vi "Monitor.vi"() -> ()   [LabVIEW 2018]
uses:
  Global Variables.vi
  <vilib>/Utility/file.llb/Read Delimited Spreadsheet (string).vi
  <vilib>/LVH/i3 JSON/i3-json.lvlib
panel:
  out "String":string
  out "Last Event":string="2:29:04 PM"
  out "Sensors Info":T1(array[cluster])
  out "Instruments":T2(array[cluster])=[{"Name"="Chassis_Sensors.vi", "vi reference"=refnum, "Running?"=FALSE}, {"Name"="PIMAX_1.vi", "vi reference"=refnum, "Running?"=FALSE}, {"Name"="PIMAX_2.vi", "vi reference"=refnum, "Running?"=FALSE}, {"Name"="MotorControl.vi", "vi reference"=refnum, "Running?"=FALSE}, {"Name"="Powermeter_library.lvlib:LV Demo Main.vi", "vi reference"=refnum, "Running?"=FALSE}, {"Name"="Multiplexer.vi", "vi reference"=refnum, "Running?"=FALSE}, {"Name"="NIR.vi", "vi reference"=refnum, "Running?"=FALSE}, {"Name"="Vis.vi", "vi reference"=refnum, "Running?"=FALSE}]
  in  "Add Custom Event":bool
  in  "Custom Event Str":string
  in  "Ring":u16(ring) items=["Proj_VaporTubes", "Proj_H2DT", "Proj_H2DT"]
  in  "Global File Information":T3={"Ring"=0, "SubFolder"="Temp Dependence", "Filename (Meas. Description)"="300C", "Measurement index"=5} {"Ring" items=["Proj_VaporTubes", "Proj_H2DT", "Proj_H2DT"]}
  out "File Size (Mb)":dbl[](array[numeric])
  in  "stop":bool
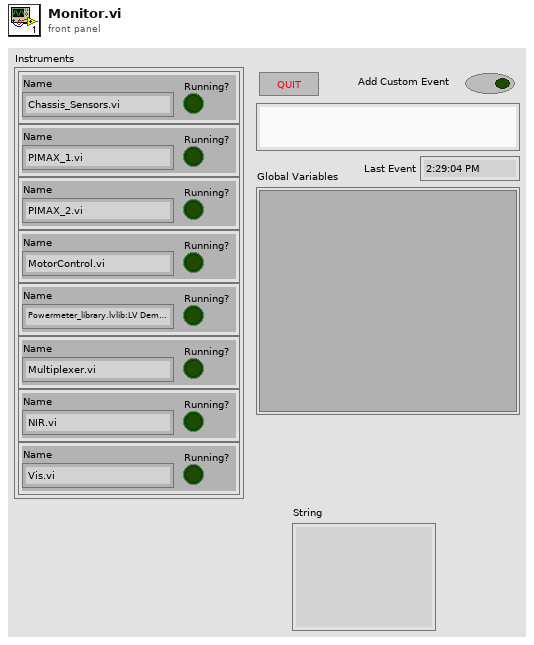
[diagram p1: front panel]
types:
  T1 = cluster{"Label.Text":string, "Panel Ref Out":refnum<vi>, bool}[]
  T2 = cluster{"Name":string, "vi reference":refnum<vi>, "Running?":bool}[]
  T3 = cluster{"Ring":u16, "SubFolder":string, "Filename (Meas. Description)":string, "Measurement index":i32}
  T4 = enum32{"Bad", "Idle", "Run top level", "Running"}
  T5 = cluster{"Name":string, "vi reference":refnum<vi>, bool}
  T6 = cluster{"Name":string, "vi reference":refnum<vi>, bool}[]
  T7 = cluster{"Project":u16, "SubFolder":string, "Filename (Meas. Description)":string, "Measurement index":i32}
  T8 = cluster{"Project 2":u16, "SubFolder 2":string, "Meas. Description 2":string, "Measurement number 2":i32}
  T9 = cluster{"Label.Text":bool, "Panel Ref Out":bool, bool}[]
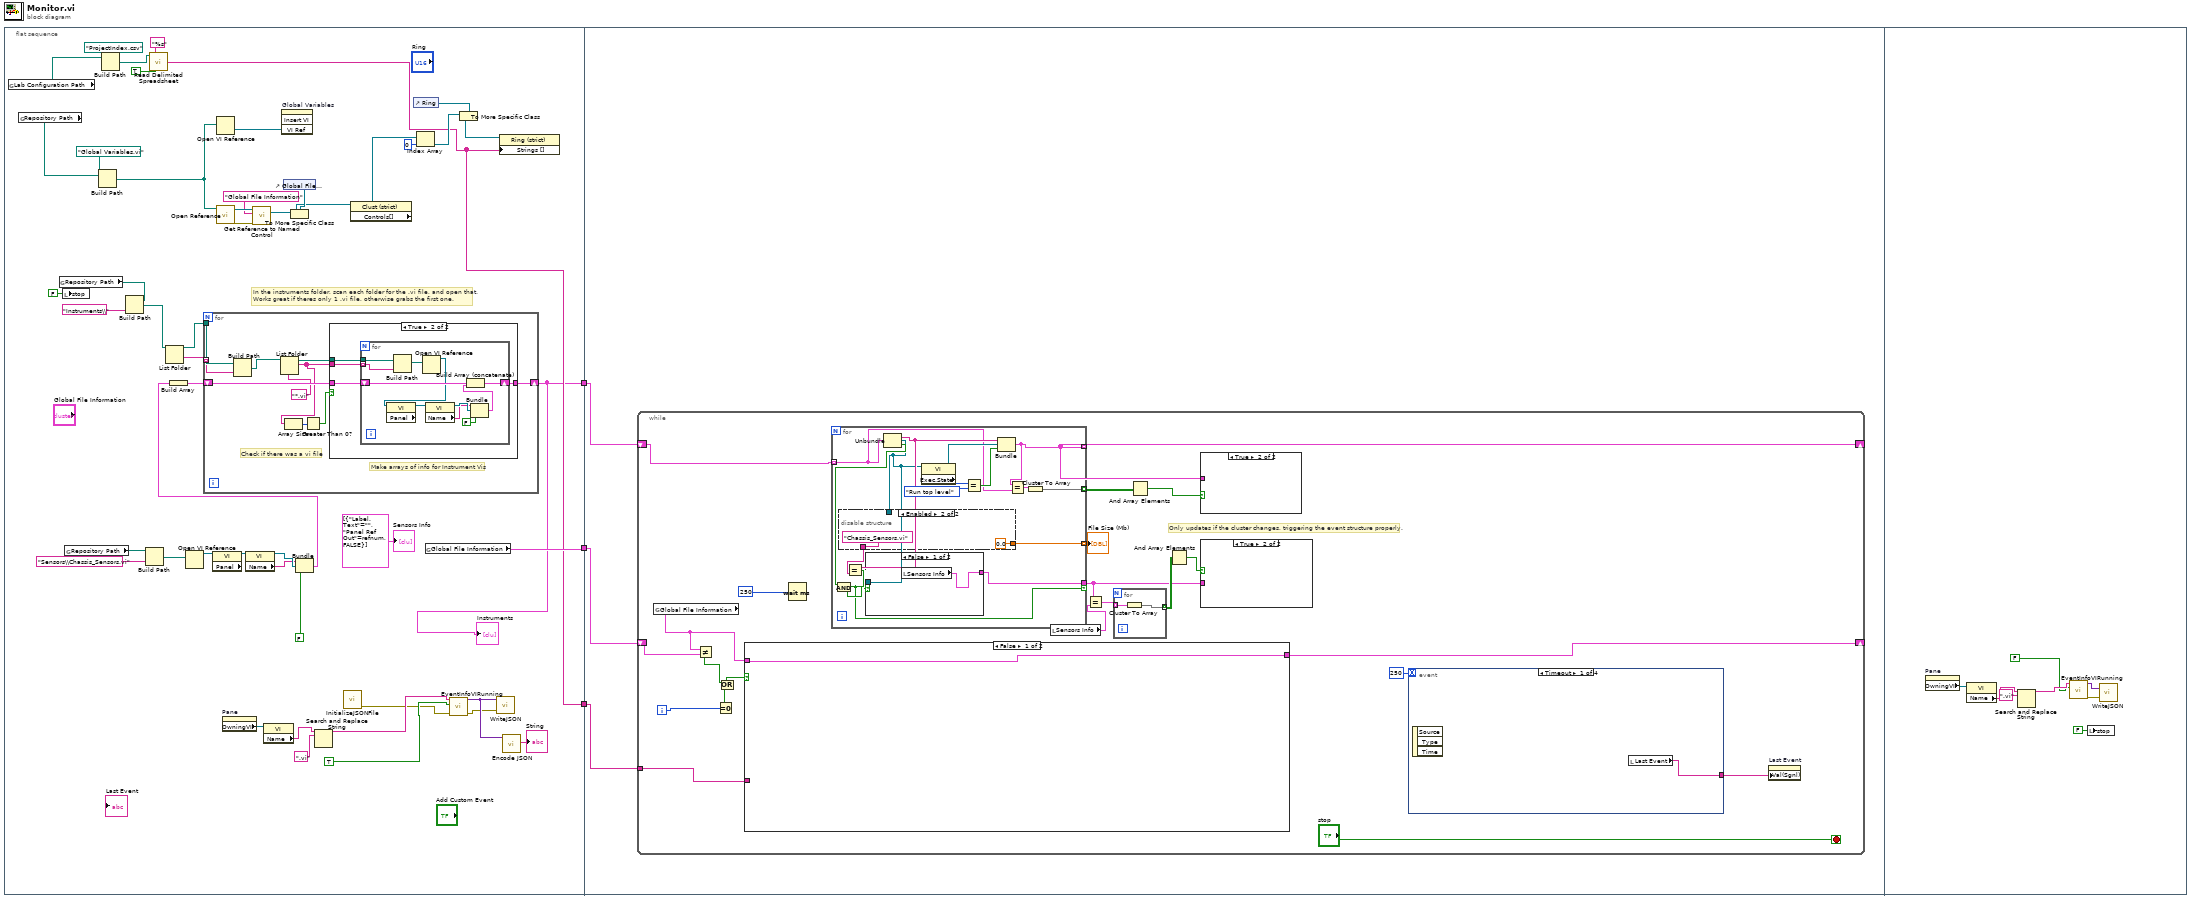
[diagram p0: block diagram]
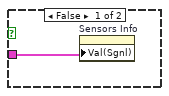
[diagram p3: hidden frame]
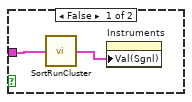
[diagram p4: hidden frame]
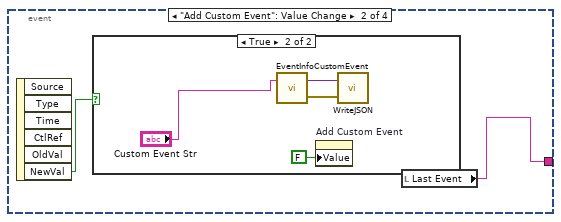
[diagram p5: hidden frame]
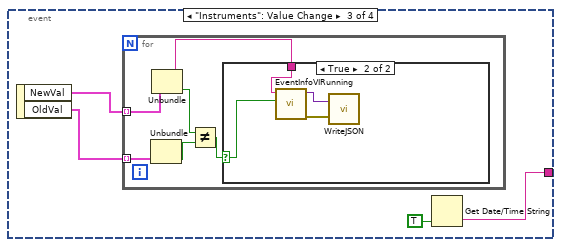
[diagram p7: hidden frame]
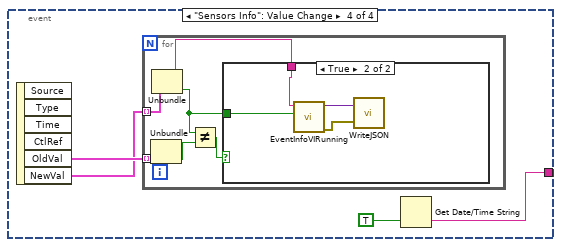
[diagram p9: hidden frame]
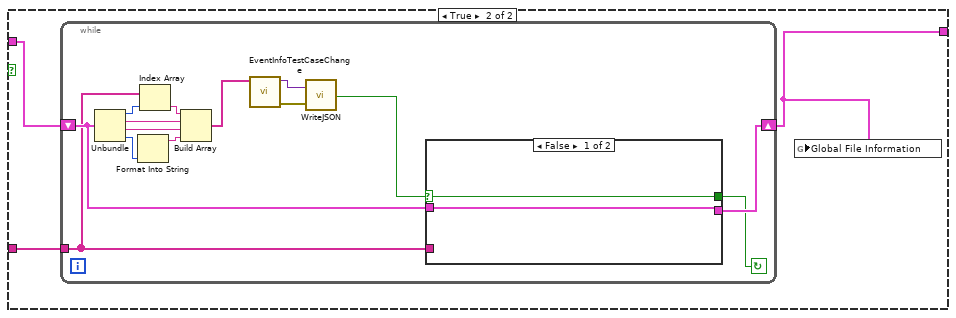
[diagram p11: hidden frame]
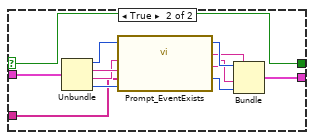
[diagram p12: hidden frame]
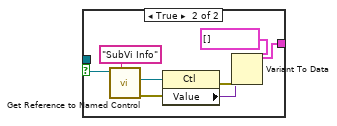
[diagram p13: hidden frame]
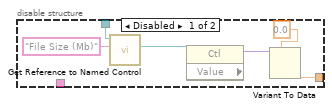
[diagram p14: hidden frame]
diagram:
  n1 = flat-sequence {
    tunnel: [w33] -> w3
    tunnel: [w10] -> w2
    tunnel: [w31] -> w1
    tunnel: w3 -> [w81]
    tunnel: w2 -> [w80]
    tunnel: w1 -> [w79]
    frame #0 {
      # "In the instruments folder, scan each folder for the .vi file, and open that.\nWorks great if theres only 1 .vi file, otherwise grabs the first one."
      n2 = global read "Global Variables.vi" "Lab Configuration Path"() -> (w11:path)
      n3 = global read "Global Variables.vi" "Repository Path"() -> (w32:path)
      n4 = global read "Global Variables.vi" "Repository Path"() -> (w27:path)
      n5 = local write "stop"(FALSE ("stop")) -> ()
      n6 = global read "Global Variables.vi" "Repository Path"() -> (w22:path)
      n7 = Build Path(base path=w32, name or relative path=path "Global Variables.vi" ("vi path")) -> (appended path=w46:path)
      n8 = Build Path(base path=w11, name or relative path=path "ProjectIndex.csv" ("vi path")) -> (appended path=w34:path)
      n9 = Build Path(base path=w27, name or relative path="Instruments\\") -> (appended path=w25:path)
      n10 = Build Path(base path=w22, name or relative path="Sensors\\Chassis_Sensors.vi") -> (appended path=w20:path)
      n11 = call-poly <vilib>:"Read Delimited Spreadsheet.vi"("file path (dialog if empty)"=w34, "format (%s)"="%s", "transpose? (F)"=TRUE) -> ("first row"=w31:string[])  [unwired: 7 in, 5 out]
      n12 = List Folder(path=w25) -> (path out=w23:path, folder names=w24:string[])  [unwired: 3 in, 2 out]
      n13 = Open VI Reference(vi path=w20) -> (vi reference=w15:refnum<vi>)  [unwired: 5 in, 1 out]
      n14 = property class="VI" props=["Panel"](reference=w15) -> (reference out=w19:refnum<vi>)  [unwired: 1 in, 2 out]
      n15 = call "Open Reference.vi"("vi path"=w46) -> ("error out"=w47:errorcluster, "Front Panel Reference"=w48:refnum<vi>)  [unwired: 5 in]
      n16 = Open VI Reference(vi path=w46) -> (vi reference=w52:refnum<vi>)  [unwired: 5 in, 1 out]
      n17 = property on="Pane" class="Pane"() -> ("OwningVI"=w30:refnum<vi>)  [unwired: 2 in, 2 out]
      n18 = property class="VI"(reference=w19) -> (reference out=w18:refnum<vi>, "Name"=w16:string)  [unwired: 1 in, 1 out]
      n19 = call "Get Reference to Named Control.vi"("error in (no error)"=w47, "Control Name"="Global File Information", "Front Panel Ref"=w48) -> ("Ctl Refnum"=w44:refnum<vi>)  [unwired: 6 in, 2 out]
      n20 = property class="VI"(reference=w30) -> ("Name"=w29:string)  [unwired: 1 in, 2 out]
      n21 = invoke on="Global Variables" class="SubPnl" method="Insert VI"("VI Ref"=w52) -> ()  [unwired: 3 in, 4 out]
      n22 = control-ref of="Global File Information"() -> (w43:refnum<vi>)
      n23 = To More Specific Class(target class=w43, reference=w44) -> (specific class reference=w42:refnum<vi>)  [unwired: 1 in, 1 out]
      n24 = Bundle("Name"=w16, "vi reference"=w18, FALSE) -> (w14:T5)  [unwired: 1 in]
      n25 = Build Array(w14) -> (w13:T6)
      n26 = for {
        shift-right: [w61] -> w10
        shift-left: w13 -> [w62]
        tunnel: w23 -> [w60]
        tunnel: w24 -> [w59] mode=indexing
        # "Check if there was a vi file"
        # "Make arrays of info for Instrument Vis"
        n27 = Build Path(base path=w60, name or relative path=w59) -> (appended path=w57:path)
        n28 = List Folder(path=w57, pattern="*.vi") -> (path out=w56:path, filenames=w55:string[])  [unwired: 2 in, 2 out]
        n29 = Array Size(array=w55) -> (size(s)=w54:i32)
        n30 = Greater Than 0?(x=w54) -> (x > 0?=w53:bool)
        n31 = case shown="True" w53 {
          tunnel: w62 -> [w63 w67]
          tunnel: [w63 w66] -> w61
          tunnel: w55 -> [_ w65]
          tunnel: w56 -> [_ w64]
          frame False {
          }
          frame True {
            n32 = for {
              tunnel: w65 -> [w68] mode=indexing
              tunnel: w64 -> [w70]
              shift-right: [w77] -> w66
              shift-left: w67 -> [w78]
              n33 = Build Path(base path=w70, name or relative path=w68) -> (appended path=w71:path)
              n34 = Open VI Reference(vi path=w71) -> (vi reference=w75:refnum<vi>)  [unwired: 5 in, 1 out]
              n35 = property class="VI" props=["Panel"](reference=w75) -> (reference out=w74:refnum<vi>)  [unwired: 1 in, 2 out]
              n36 = property class="VI"(reference=w74) -> (reference out=w73:refnum<vi>, "Name"=w69:string)  [unwired: 1 in, 1 out]
              n37 = Bundle("Name"=w69, "vi reference"=w73, FALSE) -> (w76:T5)  [unwired: 1 in]
              n38 = Build Array (concatenate)(w78, w76) -> (w77:T6)
            }
          }
        }
      }
      "Instruments" <- w10
      n39 = Search and Replace String(input string=w29, search string=".vi") -> (result string=w9:string)  [unwired: 6 in, 3 out]
      n40 = call "InitializeJSONFile.vi"() -> ("error out"=w5:errorcluster)  [unwired: 3 in, 1 out]
      n41 = property class="Clust (strict)"(reference=w42) -> ("Controls[]"=w41:refnum<vi>[])  [unwired: 1 in, 2 out]
      n42 = control-ref of="Ring"() -> (w39:refnum<vi>)
      n43 = Index Array(array=w41, index=0) -> (element=w38:refnum<vi>)
      n44 = global read "Global Variables.vi" "Global File Information"() -> (w33:T7)
      n45 = call "EventInfoVIRunning.vi"("error in (no error)"=w5, "OnOff"=TRUE, "name"=w9) -> ("error out"=w4:errorcluster, "eventinfoJSON"=w7:variant)  [unwired: 7 in]
      n46 = To More Specific Class(target class=w39, reference=w38) -> (specific class reference=w37:refnum<vi>)  [unwired: 1 in, 1 out]
      n47 = call "WriteJSON.vi"("error in (no error)"=w4, "JSONEventInfo"=w7) -> ()  [unwired: 1 in, 1 out]
      n48 = property class="Ring (strict)"(reference=w37, "Strings []"=w31) -> ()  [unwired: 1 in, 2 out]
      n49 = call <vilib>:"Encode JSON.vi"("JSON Tree"=w7) -> ("String"=→"String":string)  [unwired: 5 in, 1 out]
      "Sensors Info" <- T1 [{"Label.Text"="", "Panel Ref Out"=refnum, FALSE}] ("Sensors Info")
    }
    frame #1 {
      n50 = while {
        shift-right: [w95] -> _
        shift-left: w81 -> [w96]
        shift-right: [w91] -> _
        shift-left: w80 -> [w82]
        tunnel: w79 -> [w93]
        i -> [w99]
        stop <- "stop" stop-if-true
        # "Only updates if the cluster changes, triggering the event structure properly."
        n51 = global read "Global Variables.vi" "Global File Information"() -> (w98:T7)
        n52 = Not Equal?(x=w98, y=w96) -> (x != y?=w101:bool)
        n53 = Equal To 0?(x=w99) -> (x = 0?=w102:bool)
        n54 = Or(x=w101, y=w102) -> (x .or. y?=w97:bool)
        n55 = case shown="False" w97 {
          tunnel: w98 -> [w144 w147]
          tunnel: [w144 w146] -> w95
          tunnel: w93 -> [_ w145]
          frame False {
          }
          frame True {
            n56 = while {
              shift-right: [w156] -> w146
              shift-left: w147 -> [w157]
              tunnel: w145 -> [w154]
              stop <- w155 continue-if-true
              n57 = Unbundle(w157) -> ("Project"=w153:u16, "SubFolder"=w160:string, "Filename (Meas. Description)"=w159:string, "Measurement index"=w161:i32)
              n58 = Format Into String(w161) -> (resulting string=w158:string)  [unwired: 3 in, 1 out]
              n59 = Index Array(array=w154, index=w153) -> (element=w152:string)
              n60 = Build Array(w152, w160, w159, w158) -> (w150:string[])
              n61 = call "EventInfoTestCaseChange.vi"("TestCaseInfo"=w150) -> ("error out"=w148:errorcluster, "JSON Tree out (JSON Object)"=w149:variant)  [unwired: 9 in]
              n62 = call "WriteJSON.vi"("error in (no error)"=w148, "JSONEventInfo"=w149) -> ("test case exists?"=w151:bool)  [unwired: 1 in]
              n63 = case shown="False" w151 {
                selector: w151 -> [w162 w165]
                tunnel: w157 -> [w163 w175]
                tunnel: [w163 w166] -> w156
                tunnel: [w162 w165] -> w155
                tunnel: w154 -> [_ w164]
                frame False {
                }
                frame True {
                  n64 = Unbundle(w175) -> ("Project"=w174:u16, "SubFolder"=w173:string, "Filename (Meas. Description)"=w172:string, "Measurement index"=w171:i32)
                  n65 = call "Prompt_EventExists.vi"("Project Strings"=w164, "Measurement number"=w171, "Meas. Description"=w172, "SubFolder"=w173, "Project"=w174) -> ("Meas. Description 2"=w168:string, "SubFolder 2"=w169:string, "Project 2"=w170:u16, "Measurement number 2"=w167:i32)  [unwired: 1 in]
                  n66 = Bundle("Project 2"=w170, "SubFolder 2"=w169, "Meas. Description 2"=w168, "Measurement number 2"=w167) -> (w166:T8)  [unwired: 1 in]
                }
              }
            }
            n67 = global write "Global Variables.vi" "Global File Information"(w146) -> ()
          }
        }
        n68 = Wait (ms)(milliseconds to wait=250 ("Wait time (ms)")) -> ()  [unwired: 1 out]
        n69 = for {
          tunnel: w82 -> [w182] mode=indexing
          tunnel: [w183] -> w91 mode=indexing
          tunnel: [w189] -> w94 mode=indexing
          tunnel: [w178] -> w85 if=w176
          tunnel: [w180] -> w90 mode=indexing
          n70 = Unbundle(w182) -> ("Name"=w185:string, "vi reference"=w184:refnum<vi>, w186:bool)
          n71 = disable-structure shown="Enabled" {
            disable-tunnel: [w204 0.0] -> w189
            disable-tunnel: w184 -> [w203 _]
            disable-tunnel: [_ "Chassis_Sensors.vi"] -> w177
            frame Disabled {
              n72 = call "Get Reference to Named Control.vi"("Control Name"="File Size (Mb)", "Front Panel Ref"=w203) -> ("Ctl Refnum"=w201:refnum<vi>)  [unwired: 7 in, 2 out]
              n73 = property class="Ctl"(reference=w201) -> ("Value"=w206:variant)  [unwired: 1 in, 2 out]
              n74 = Variant To Data(type=0.0, Variant=w206) -> (data=w204:dbl)  [unwired: 1 in, 1 out]
            }
            frame Enabled {
            }
          }
          n75 = Equal?(x=w185, y=w177) -> (x = y?=w179:bool)
          n76 = And(x=w186, y=w179) -> (x .and. y?=w176:bool)
          n77 = case shown="False" w176 {
            tunnel: w184 -> [_ w200]
            tunnel: [w192 w193] -> w178
            frame False {
              n78 = local read "Sensors Info"() -> (w192:T1)
            }
            frame True {
              n79 = call "Get Reference to Named Control.vi"("Control Name"="SubVi Info", "Front Panel Ref"=w200) -> ("error out"=w197:errorcluster, "Ctl Refnum"=w198:refnum<vi>)  [unwired: 7 in, 1 out]
              n80 = property class="Ctl"(reference=w198, error in=w197) -> (error out=w196:errorcluster, "Value"=w195:variant)  [unwired: 1 out]
              n81 = Variant To Data(error in=w196, type=T1 [] ("Subvi Info"), Variant=w195) -> (data=w193:T1)  [unwired: 1 out]
            }
          }
          n82 = property class="VI"(reference=w184) -> (reference out=w188:refnum<vi>, "Exec.State"=w191:T4)  [unwired: 1 in, 1 out]
          n83 = Equal?(x=w191, y=T4."Run top level" ("Execution:State 2")) -> (x = y?=w187:bool)
          n84 = Bundle("Name"=w185, "vi reference"=w188, w187) -> (w183:T5)  [unwired: 1 in]
          n85 = Equal?(x=w183, y=w182) -> (x = y?=w181:cluster{"Name":bool, "vi reference":bool, bool})
          n86 = Cluster To Array(cluster=w181) -> (array=w180:bool[])
        }
        "File Size (Mb)" <- w94
        n87 = local read "Sensors Info"() -> (w83:T1)
        n88 = Equal?(x=w85, y=w83) -> (x = y?=w84:T9)
        n89 = for {
          tunnel: w84 -> [w105] mode=indexing
          tunnel: [w104] -> w86 mode=indexing
          n90 = Cluster To Array(cluster=w105) -> (array=w104:bool[])
        }
        n91 = And Array Elements(Boolean array=w90) -> (logical AND=w89:bool)
        n92 = And Array Elements(Boolean array=w86) -> (logical AND=w87:bool)
        n93 = case shown="True" w89 {
          tunnel: w91 -> [w107 _]
          frame False {
            n94 = call "SortRunCluster.vi"("Array"=w107) -> ("output array"=w108:T6)
            n95 = property on="Instruments" class="Arr (strict)"("Val(Sgnl)"=w108) -> ()  [unwired: 2 in, 2 out]
          }
          frame True {
          }
        }
        n96 = case shown="True" w87 {
          tunnel: w85 -> [w106 _]
          frame False {
            n97 = property on="Sensors Info" class="Arr (strict)"("Val(Sgnl)"=w106) -> ()  [unwired: 2 in, 2 out]
          }
          frame True {
          }
        }
        n98 = event shown="[0] Timeout" {
          selector: _ -> [_ _ _ _]
          dyn-events: _ -> [_ _ _ _]
          timeout: 250 -> [_ _ _ _]
          tunnel: [w109 w110 w119 w131] -> w92
          event Timeout {
            n99 = event-data() -> ()  [unwired: 1 in, 3 out]
            n100 = local read "Last Event"() -> (w109:string)
          }
          event "Add Custom Event": Value Change {
            n101 = event-data() -> ("NewVal"=w111:bool)  [unwired: 1 in, 5 out]
            n102 = case shown="True" w111 {
              frame False {
              }
              frame True {
                n103 = call "EventInfoCustomEvent.vi"("eventstr"="Custom Event Str") -> ("error out"=w112:errorcluster, "JSON Tree out (JSON Object)"=w113:variant)  [unwired: 1 in]
                n104 = property on="Add Custom Event" class="Bool (strict)"("Value"=FALSE ("Add Custom Event")) -> ()  [unwired: 2 in, 2 out]
                n105 = call "WriteJSON.vi"("error in (no error)"=w112, "JSONEventInfo"=w113) -> ()  [unwired: 1 in, 1 out]
              }
            }
            n106 = local read "Last Event"() -> (w110:string)
          }
          event "Instruments": Value Change {
            n107 = event-data() -> ("NewVal"=w117:T2, "OldVal"=w118:T2)  [unwired: 1 in]
            n108 = for {
              tunnel: w117 -> [w125] mode=indexing
              tunnel: w118 -> [w123] mode=indexing
              n109 = Unbundle(w123) -> ("Running?"=w121:bool)  [unwired: 2 out]
              n110 = Unbundle(w125) -> ("Name"=w124:string, "Running?"=w120:bool)  [unwired: 1 out]
              n111 = Not Equal?(x=w120, y=w121) -> (x != y?=w122:bool)
              n112 = case shown="True" w122 {
                selector: w122 -> [_ w126]
                tunnel: w124 -> [_ w129]
                frame False {
                }
                frame True {
                  n113 = call "EventInfoVIRunning.vi"("OnOff"=w126, "name"=w129) -> ("error out"=w127:errorcluster, "eventinfoJSON"=w128:variant)  [unwired: 8 in]
                  n114 = call "WriteJSON.vi"("error in (no error)"=w127, "JSONEventInfo"=w128) -> ()  [unwired: 1 in, 1 out]
                }
              }
            }
            n115 = Get Date/Time String(want seconds? (F)=TRUE) -> (time string=w119:string)  [unwired: 2 in, 1 out]
          }
          event "Sensors Info": Value Change {
            n116 = event-data() -> ("OldVal"=w133:T1, "NewVal"=w132:T1)  [unwired: 1 in, 4 out]
            n117 = for {
              tunnel: w132 -> [w139] mode=indexing
              tunnel: w133 -> [w137] mode=indexing
              n118 = Unbundle(w137) -> (w135:bool)  [unwired: 2 out]
              n119 = Unbundle(w139) -> ("Label.Text"=w138:string, w134:bool)  [unwired: 1 out]
              n120 = Not Equal?(x=w134, y=w135) -> (x != y?=w136:bool)
              n121 = case shown="True" w136 {
                tunnel: w138 -> [_ w143]
                tunnel: w134 -> [_ w142]
                frame False {
                }
                frame True {
                  n122 = call "EventInfoVIRunning.vi"("OnOff"=w142, "name"=w143) -> ("error out"=w140:errorcluster, "eventinfoJSON"=w141:variant)  [unwired: 8 in]
                  n123 = call "WriteJSON.vi"("error in (no error)"=w140, "JSONEventInfo"=w141) -> ()  [unwired: 1 in, 1 out]
                }
              }
            }
            n124 = Get Date/Time String(want seconds? (F)=TRUE) -> (time string=w131:string)  [unwired: 2 in, 1 out]
          }
        }
        n125 = property on="Last Event" class="Str"("Val(Sgnl)"=w92) -> ()  [unwired: 2 in, 2 out]
      }
    }
    frame #2 {
      n126 = property on="Pane" class="Pane"() -> ("OwningVI"=w215:refnum<vi>)  [unwired: 2 in, 2 out]
      n127 = property class="VI"(reference=w215) -> ("Name"=w214:string)  [unwired: 1 in, 2 out]
      n128 = Search and Replace String(input string=w214, search string=".vi") -> (result string=w212:string)  [unwired: 6 in, 3 out]
      n129 = call "EventInfoVIRunning.vi"("OnOff"=FALSE, "name"=w212) -> ("error out"=w209:errorcluster, "eventinfoJSON"=w210:variant)  [unwired: 8 in]
      n130 = local write "stop"(FALSE ("stop")) -> ()
      n131 = call "WriteJSON.vi"("error in (no error)"=w209, "JSONEventInfo"=w210) -> ()  [unwired: 1 in, 1 out]
    }
  }
